vi "Close Instrument.vi"(7 "Go Local (\"@LOC\")":bool, 8 "error in (no error)":errorcluster, 11 "VNA-Keysight PNA in":refnum<class "VNA-Keysight PNA.lvclass">) -> (0 "error out":errorcluster, 3 "VNA-Keysight PNA out":refnum<class "VNA-Keysight PNA.lvclass">)   [LabVIEW 2020, in "VNA-Keysight PNA.lvclass"]
uses:
  VNA-Keysight PNA.lvclass
  C:/Sandbox/RF Bench/Source Code/WiSpry Test Framework/Instruments/Instrument.lvclass
  Instrument.lvclass/Instrument.ctl
  Vector Network Analyzer.lvclass
  Instrument.lvclass
  <instrlib>/Keysight PNA Series/Keysight PNA Series.lvlib
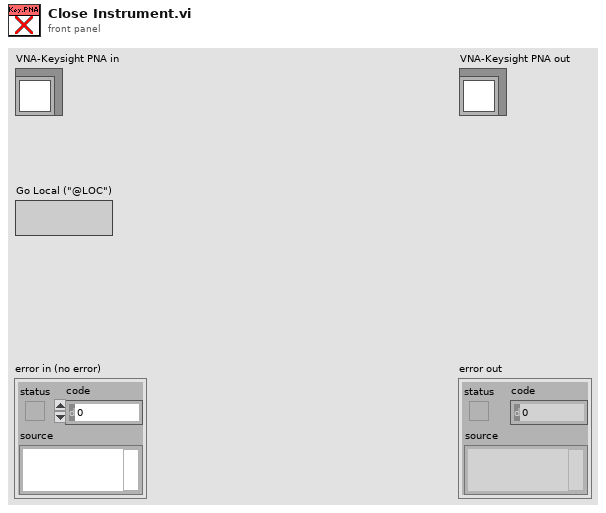
[diagram p1: front panel]
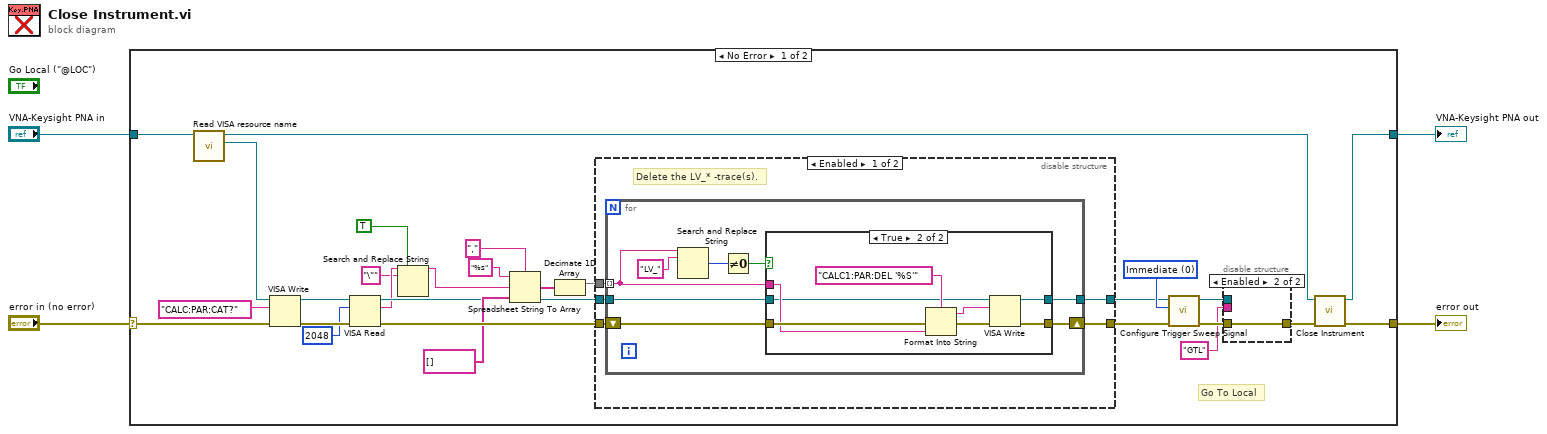
[diagram p0: block diagram]
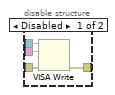
[diagram p2: hidden frame]
diagram:
  n1 = case shown="No Error" "error in (no error)" {
    selector: "error in (no error)" -> [w29 w63]
    tunnel: "VNA-Keysight PNA in" -> [w31 w62]
    tunnel: [w7 w63] -> w2
    tunnel: [w5 w62] -> w1
    frame No Error {
      w30 = 0 items=["Immediate", "External", "Manual"] ("Trigger Source (0: Immediate)")
      # "Go To Local"
      n2 = call "Read VISA resource name.vi"("Instrument in"=w31) -> ("VISA resource name"=w13:refnum<visa-resource-name>, "Instrument out"=w6:refnum<class "VNA-Keysight PNA.lvclass">)  [unwired: 9 in]
      n3 = VISA Write(VISA resource name=w13, write buffer="CALC:PAR:CAT?") -> (VISA resource name out=w26:refnum<visa-resource-name>, error out=w27:errorcluster)  [unwired: 1 in, 1 out]
      n4 = VISA Read(VISA resource name=w26, byte count=u32 2048, error in (no error)=w27) -> (VISA resource name out=w20:refnum<visa-resource-name>, read buffer=w18:string, error out=w19:errorcluster)  [unwired: 1 out]
      n5 = Search and Replace String(replace all?=TRUE ("replace all? (F)"), input string=w18, search string="\"") -> (result string=w16:string)  [unwired: 5 in, 3 out]
      n6 = Spreadsheet String To Array(delimiter (Tab)=",", format string="%s", spreadsheet string=w16, array type (2D Dbl)=string[] []) -> (array=w21:string[])
      n7 = Decimate 1D Array(w21) -> (w14:string[])  [unwired: 1 out]
      n8 = disable-structure shown="Enabled" {
        disable-tunnel: w20 -> [w41 w61]
        disable-tunnel: w19 -> [w40 w60]
        disable-tunnel: w14 -> [w39 _]
        disable-tunnel: [w38 w60] -> _
        disable-tunnel: [w37 w61] -> w12
        frame Enabled {
          # "Delete the LV_* -trace(s)."
          n9 = for {
            tunnel: w41 -> [w46]
            shift-right: [w43] -> w38
            shift-left: w40 -> [w45]
            tunnel: w39 -> [w44] mode=indexing
            tunnel: [w42] -> w37
            n10 = Search and Replace String(input string=w44, search string="LV_") -> (number of replacements=w48:i32)  [unwired: 6 in, 3 out]
            n11 = Not Equal To 0?(x=w48) -> (x != 0?=w47:bool)
            n12 = case shown="True" w47 {
              tunnel: w46 -> [w50 w55]
              tunnel: w45 -> [w51 w53]
              tunnel: w44 -> [_ w59]
              tunnel: [w51 w58] -> w43
              tunnel: [w50 w54] -> w42
              frame False {
              }
              frame True {
                n13 = Format Into String(format string="CALC1:PAR:DEL '%S'" ("string"), error in=w53, w59) -> (resulting string=w56:string, error out=w52:errorcluster)  [unwired: 1 in]
                n14 = VISA Write(VISA resource name=w55, write buffer=w56, error in (no error)=w52) -> (VISA resource name out=w54:refnum<visa-resource-name>, error out=w58:errorcluster)  [unwired: 1 out]
              }
            }
          }
        }
        frame Disabled {
          # "Don't delete the trace(s)."
        }
      }
      n15 = call <instrlib>:"Configure Trigger Sweep Signal.vi"("error in (no error)"=w29, "Trigger Source (0: Immediate)"=w30, "VISA resource name"=w12) -> ("error out"=w10:errorcluster, "VISA resource name out"=w11:refnum<visa-resource-name>)  [unwired: 7 in]
      n16 = disable-structure shown="Enabled" {
        disable-tunnel: w11 -> [w35 _]
        disable-tunnel: w10 -> [w34 w36]
        disable-tunnel: "GTL" ("write buffer") -> [w33 _]
        disable-tunnel: [w32 w36] -> w8
        frame Disabled {
          n17 = VISA Write(VISA resource name=w35, write buffer=w33, error in (no error)=w34) -> (error out=w32:errorcluster)  [unwired: 2 out]
        }
        frame Enabled {
        }
      }
      n18 = call-parent "Close Instrument.vi"("error in (no error)"=w8, "Instrument in"=w6) -> ("error out"=w7:errorcluster, "Instrument out"=w5:refnum<class "VNA-Keysight PNA.lvclass">)  [unwired: 8 in]
    }
    frame Error {
    }
  }
  "error out" <- w2
  "VNA-Keysight PNA out" <- w1
